vi "MathCad_Matrix_Get_2D.vi"(1 "Mathcad.IMatrixValue Refnum":refnum<k7>, 2 "error out 2":errorcluster) -> (4 "Mathcad.IMatrixValue Refnum":refnum<k7>, 5 "Array":variant[][](array[variant]), 6 "error out":errorcluster)   [LabVIEW 2015]
doc: "Gets the value from the reference retrieved from the getrefnum VI."
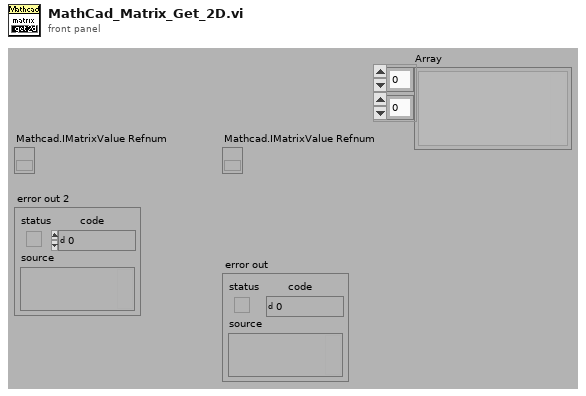
[diagram p1: front panel]
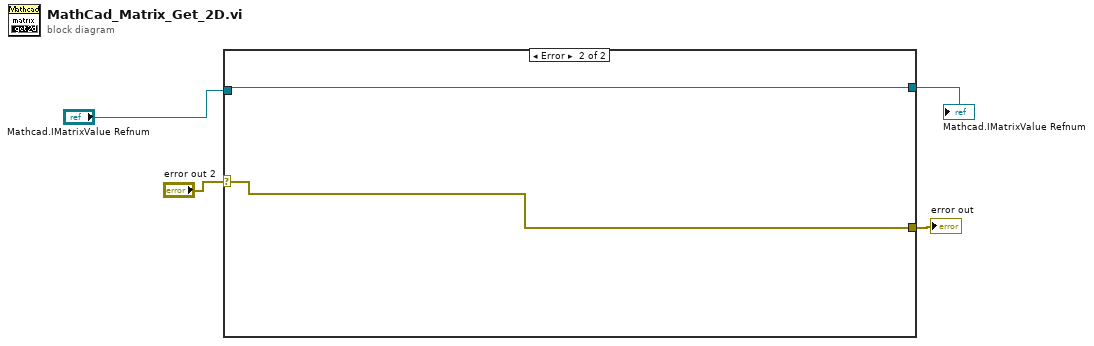
[diagram p0: block diagram]
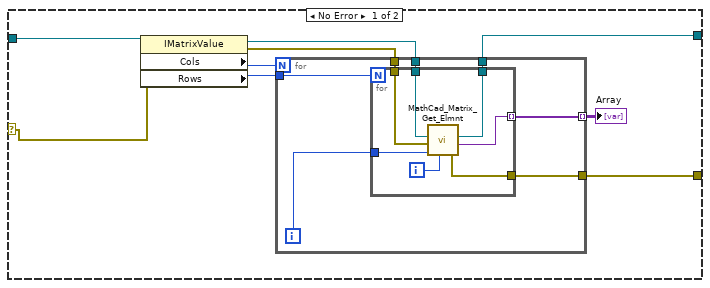
[diagram p2: hidden frame]
diagram:
  n1 = case shown="Error" "error out 2" {
    selector: "error out 2" -> [w13 w29]
    tunnel: [w6 w29] -> w3
    tunnel: "Mathcad.IMatrixValue Refnum" -> [w12 w28]
    tunnel: [w7 w28] -> w1
    frame No Error {
      n2 = property class="IMatrixValue"(reference=w12, error in=w13) -> (reference out=w9:refnum<k7>, error out=w8:errorcluster, "Cols"=w11:i32, "Rows"=w10:i32)
      n3 = for {
        N: w11 -> [_]
        tunnel: w10 -> [w20]
        tunnel: [w18] -> w5 mode=indexing
        tunnel: w9 -> [w17]
        tunnel: w8 -> [w16]
        tunnel: [w15] -> w7
        tunnel: [w14] -> w6
        i -> [w19]
        n4 = for {
          N: w20 -> [_]
          tunnel: w19 -> [w27]
          tunnel: [w21] -> w18 mode=indexing
          tunnel: w17 -> [w25]
          tunnel: w16 -> [w24]
          tunnel: [w23] -> w15
          tunnel: [w22] -> w14
          i -> [w26]
          n5 = call "MathCad_Matrix_Get_Elmnt.vi"("row"=w26, "col"=w27, "error in"=w24, "Mathcad.IMatrixValue Refnum"=w25) -> ("error out"=w22:errorcluster, "GetElement"=w21:variant, "Mathcad.IMatrixValue Refnum"=w23:refnum<k7>)  [unwired: 3 in]
        }
      }
      "Array" <- w5
    }
    frame Error {
    }
  }
  "Mathcad.IMatrixValue Refnum" <- w1
  "error out" <- w3
